vi "隐藏页面.vi"(0 "主选项卡":enum32{"自动", "手动", "设置", "校准"}(ring)=enum."设置", 1 "TabControl输入":refnum<vi>) -> ()   [LabVIEW 2014]
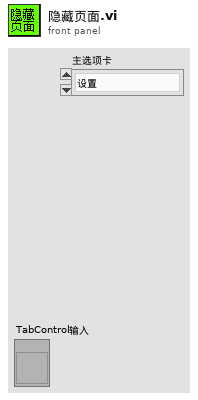
[diagram p1: front panel]
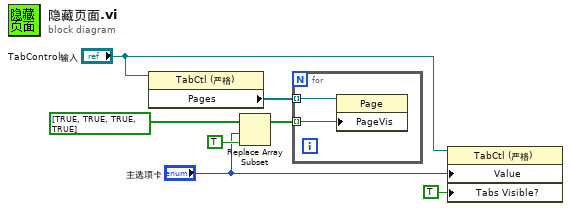
[diagram p0: block diagram]
diagram:
  n1 = property class="TabCtl (严格)"(reference="TabControl输入") -> ("Pages"=w7:refnum<vi>[])  [unwired: 1 in, 2 out]
  n2 = Replace Array Subset(array=bool[] [TRUE, TRUE, TRUE, TRUE], new element=TRUE ("新元素/子数组"), index="主选项卡") -> (w4:bool[])
  n3 = for {
    tunnel: w7 -> [w9] mode=indexing
    tunnel: w4 -> [w8] mode=indexing
    n4 = property class="Page"(reference=w9, "PageVis"=w8) -> ()  [unwired: 1 in, 2 out]
  }
  n5 = property class="TabCtl (严格)"(reference="TabControl输入", "Value"="主选项卡", "Tabs Visible?"=TRUE ("选项卡可见？")) -> ()  [unwired: 1 in, 2 out]
